vi "Serial no.vi"(11 "Serial no":string) -> (3 "String":string)   [LabVIEW 2015]
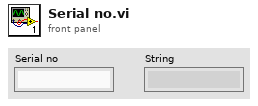
[diagram p1: front panel]
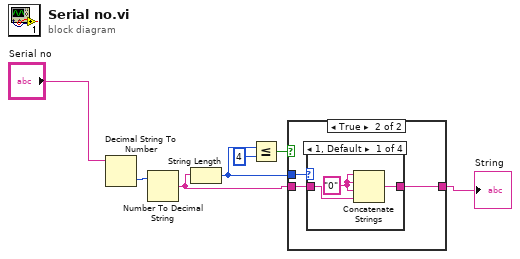
[diagram p0: block diagram]
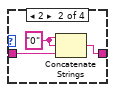
[diagram p3: hidden frame]
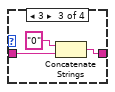
[diagram p4: hidden frame]
diagram:
  n1 = Decimal String To Number(string="Serial no") -> (number=w1:i32)  [unwired: 2 in, 1 out]
  n2 = Number To Decimal String(number=w1) -> (decimal integer string=w5:string)  [unwired: 1 in]
  n3 = String Length(string=w5) -> (length=w3:i32)
  n4 = Less Or Equal?(x=w3, y=4) -> (x <= y?=w2:bool)
  n5 = case shown="True" w2 {
    tunnel: w3 -> [_ w10]
    tunnel: w5 -> [_ w9]
    tunnel: [_ w8] -> w7
    frame False {
    }
    frame True {
      n6 = case shown="1, Default" w10 {
        tunnel: w9 -> [w12 w14 w18 w20]
        tunnel: [w11 w15 w17 w20] -> w8
        frame 1, Default {
          w13 = "0" ("string")
          n7 = Concatenate Strings(w13, w13, w13, w12) -> (w11:string)
        }
        frame 2 {
          w16 = "0" ("string")
          n8 = Concatenate Strings(w16, w16, w14) -> (w15:string)
        }
        frame 3 {
          n9 = Concatenate Strings("0" ("string"), w18) -> (w17:string)
        }
        frame 4 {
        }
      }
    }
  }
  "String" <- w7
